vi "Add_Shear_Ramp_Step_Job.vi"(7 "New Job":bool=TRUE, 8 "error in (no error)":errorcluster, 9 "Tag Item":string, 10 "ShearRampStepConfiguration":T1={"Rotation or Torque"="Rotation (RPM)", "Initial Value"=0.0, "Final Value"=0.0, "Step Duration"=0.0, "Number of Steps"=0, "Shear Ramp Step Array"=[], "Confirmed?"=FALSE, "Shear Step Generation"=enum."StepDurationConstant"}, 11 "TreeControl in":refnum<vi>) -> (0 "error out":errorcluster)   [LabVIEW 2021]
uses:
  TypeDefs/ShearRampStepConfiguration.ctl
panel:
  out "TreeControl out":refnum<vi>
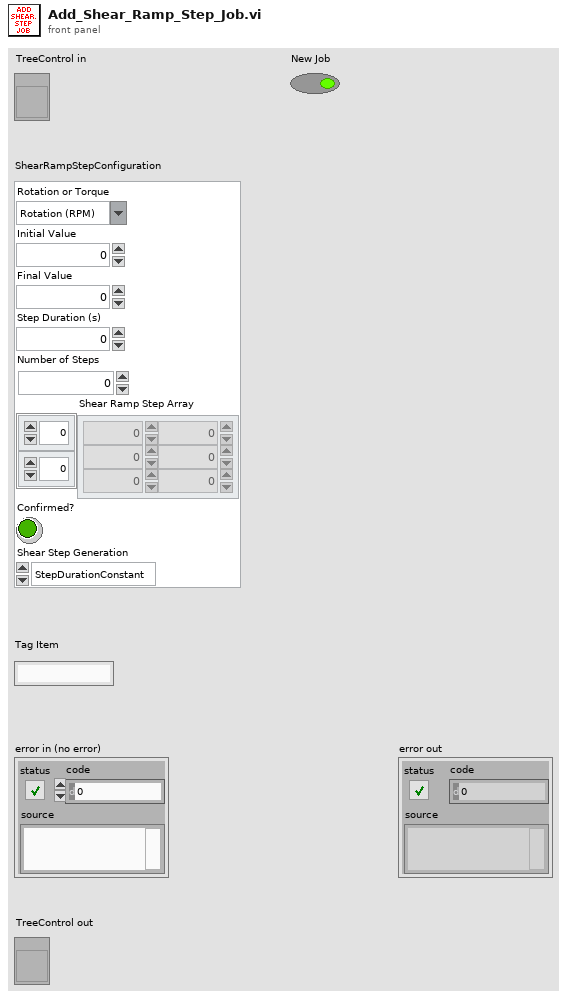
[diagram p1: front panel]
types:
  T1 = typedef "ShearRampStepConfiguration.ctl" = cluster{"Rotation or Torque":string, "Initial Value":dbl, "Final Value":dbl, "Step Duration":dbl, "Number of Steps":i32, "Shear Ramp Step Array":dbl[][], "Confirmed?":bool, "Shear Step Generation":enum16{"StepDurationConstant", "Table"}}
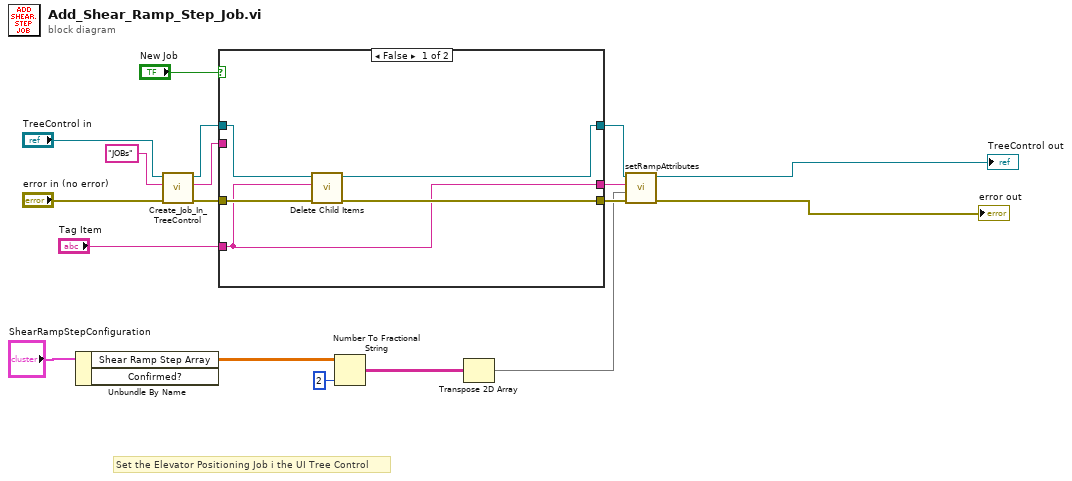
[diagram p0: block diagram]
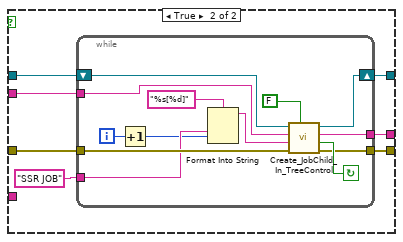
[diagram p2: hidden frame]
diagram:
  # "Set the Elevator Positioning Job i the UI Tree Control"
  n1 = Unbundle By Name("ShearRampStepConfiguration") -> ("Shear Ramp Step Array"=w12:dbl[][])  [unwired: 1 out]
  n2 = call "Create_Job_In_TreeControl.vi"("error in (no error)"="error in (no error)", "Left Cell String"="JOBs", "TreeControl in"="TreeControl in") -> ("error out"=w14:errorcluster, "Edit Tree Items:Add Item"=w17:string, "TreeControl out"=w18:refnum<vi>)  [unwired: 6 in]
  n3 = case shown="False" "New Job" {
    tunnel: w18 -> [w22 w30]
    tunnel: w17 -> [_ w29]
    tunnel: w14 -> [w23 w27]
    tunnel: [w19 w26] -> w11
    tunnel: [w20 w25] -> w10
    tunnel: [w21 w24] -> w8
    tunnel: "Tag Item" -> [w19 _]
    frame False {
      n4 = call "Delete Child Items.vi"("error in (no error)"=w23, "Item Edit"=w19, "TreeControl in"=w22) -> ("error out"=w20:errorcluster, "TreeControl out"=w21:refnum<vi>)  [unwired: 7 in]
    }
    frame True {
      n5 = while {
        tunnel: w27 -> [w43]
        tunnel: "SSR JOB" -> [w32]
        tunnel: w29 -> [w40]
        tunnel: [w35] -> w25
        tunnel: [w34] -> w26
        shift-right: [w33] -> w24
        shift-left: w30 -> [w39]
        i -> [w37]
        stop <- w36 continue-if-true
        n6 = Increment(x=w37) -> (x+1=w31:i32)
        n7 = Format Into String(format string="%s[%d]", w32, w31) -> (resulting string=w41:string)  [unwired: 2 in, 1 out]
        n8 = call "Create_JobChild_In_TreeControl.vi"("Child Only?"=FALSE, "error in (no error)"=w43, "Child Tag Name"=w41, "Parent Item"=w40, "TreeControl in"=w39) -> ("error out"=w35:errorcluster, "Tag Already Exists?"=w36:bool, "Edit Tree Items:Add Item 2"=w34:string, "TreeControl out"=w33:refnum<vi>)  [unwired: 3 in]
      }
    }
  }
  n9 = Number To Fractional String(number=w12, precision (6)=i16 2) -> (F-format string=w4:string[][])  [unwired: 2 in]
  n10 = Transpose 2D Array(2D array=w4) -> (transposed array=w3:string[][])
  n11 = call "setRampAttributes.vi"("error in (no error)"=w10, "Array"=w3, "Edit Tree Items:Add Item in"=w11, "TreeControl in"=w8) -> ("error out"=→"error out":errorcluster, "TreeControl out"=→"TreeControl out":refnum<vi>)  [unwired: 6 in]
